vi "PR4000 cfg range.vi"(10 "Channel parsed command info":T1, 11 "MKS4000b in":refnum<class "MKS4000b.lvclass">) -> (2 "new commands":string, 3 "MKS4000b out":refnum<class "MKS4000b.lvclass">)   [LabVIEW 2020, in "MKS4000b.lvclass"]
uses:
  MKS4000b.lvclass
  channel parsed cmd cluster.ctl
  MKS4000b.lvclass/MKS4000b.ctl
  CompressAndUpdate(Numeric).vi
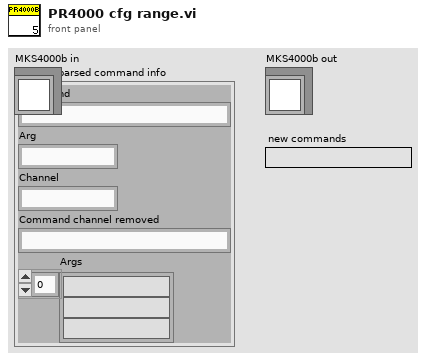
[diagram p1: front panel]
types:
  T1 = typedef "channel parsed cmd cluster.ctl" = cluster{"Command":string, "Arg":string, "Channel":string, "Command channel removed":string, "Args":string[]}
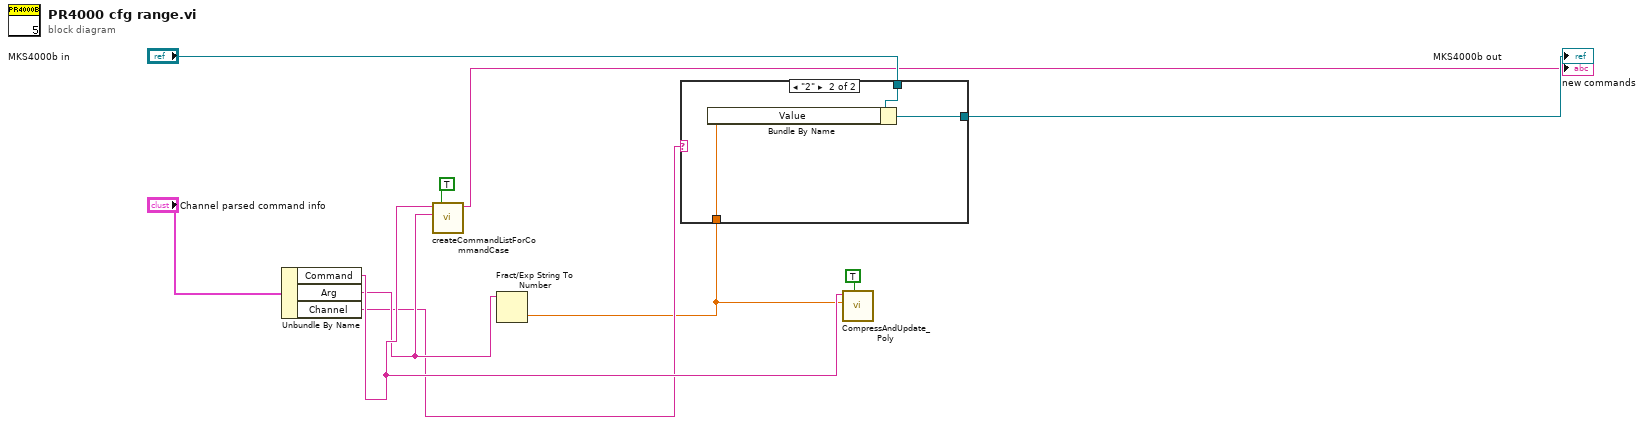
[diagram p0: block diagram]
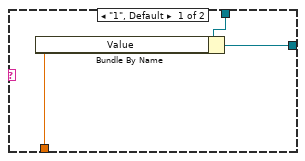
[diagram p2: hidden frame]
diagram:
  n1 = Unbundle By Name("Channel parsed command info") -> ("Command"=w10:string, "Arg"=w9:string, "Channel"=w7:string)
  n2 = call "createCommandListForCommandCase.vi"("immediate Check (only once)"=TRUE, "setvalue"=w9, "command"=w10) -> ("new commands"=→"new commands":string)  [unwired: 8 in]
  n3 = Fract/Exp String To Number(string=w9) -> (number=w6:dbl)  [unwired: 3 in, 1 out]
  n4 = case shown="\"2\"" w7 {
    tunnel: "MKS4000b in" -> [w13 w16]
    tunnel: [w12 w15] -> w4
    tunnel: w6 -> [w11 w14]
    frame "1", Default {
      n5 = Bundle By Name(cluster=w13, "Value"=w11) -> (w12:refnum<class "MKS4000b.lvclass">)
    }
    frame "2" {
      n6 = Bundle By Name(cluster=w16, "Value"=w14) -> (w15:refnum<class "MKS4000b.lvclass">)
    }
  }
  "MKS4000b out" <- w4
  n7 = call-poly "CompressAndUpdate_Poly.vi"("force CVT update (false)"=TRUE ("force CVT update"), "Numeric"=w6, "command or variable name"=w10) -> ()  [unwired: 8 in, 1 out]
